vi "Init TS DAC Results File.vi"(8 "error in":errorcluster, 11 "Generic Test Stand in":refnum<class "Generic Test Stand.lvclass">) -> (0 "error out":errorcluster, 3 "Generic Test Stand out":refnum<class "Generic Test Stand.lvclass">)   [LabVIEW 2019, in "Generic Test Stand.lvclass"]
uses:
  Generic Test Stand.lvclass
  Generic Test Stand.lvclass/Generic Test Stand.ctl
  DAC/DAC.lvclass
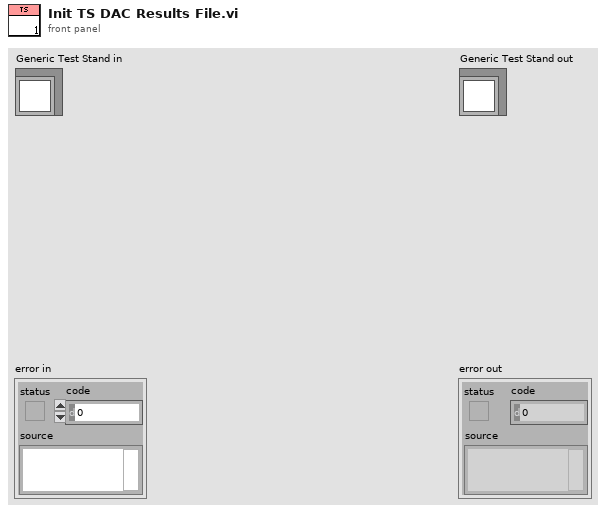
[diagram p1: front panel]
types:
  T1 = enum16{"open", "open or create", "create or replace", "create", "open (read-only)"}
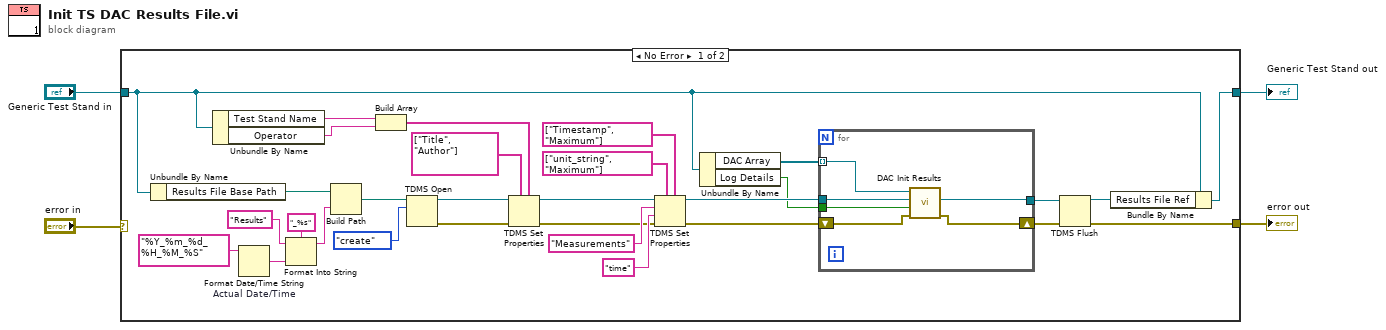
[diagram p0: block diagram]
diagram:
  n1 = case shown="No Error" "error in" {
    selector: "error in" -> [_ w42]
    tunnel: [w30 w42] -> w1
    tunnel: [w33 w41] -> w2
    tunnel: "Generic Test Stand in" -> [w21 w41]
    frame No Error {
      n2 = Unbundle By Name(w21) -> ("Results File Base Path"=w29:path)
      n3 = Unbundle By Name(w21) -> ("Test Stand Name"=w20:string, "Operator"=w19:string)
      n4 = Format Date/Time String "Actual Date/Time"(time format string (%c)="%Y_%m_%d_%H_%M_%S") -> (date/time string=w26:string)  [unwired: 2 in]
      n5 = Format Into String(format string="_%s", initial string="Results", w26) -> (resulting string=w24:string)  [unwired: 1 in, 1 out]
      n6 = Build Path(base path=w29, name or relative path=w24) -> (appended path=w23:path)
      n7 = Build Array(w20, w19) -> (w16:string[])
      n8 = TDMS Open(10:T1."create" ("operation (0:open)"), 11:w23) -> (0:w15:errorcluster, 3:w18:refnum<k34>)  [unwired: 5 in]
      n9 = TDMS Set Properties(5:w16, 7:string[] ["Title", "Author"] ("property names"), 8:w15, 11:w18) -> (0:w9:errorcluster, 3:w10:refnum<k34>)  [unwired: 2 in, 2 out]
      n10 = TDMS Set Properties(5:string[] ["Timestamp", "Maximum"] ("property names"), 7:string[] ["unit_string", "Maximum"] ("property names"), 8:w9, 9:"time" ("channel name"), 10:"Measurements" ("group name in (Untitled)"), 11:w10) -> (0:w8:errorcluster, 3:w7:refnum<k34>)  [unwired: 2 out]
      n11 = Unbundle By Name(w21) -> ("DAC Array"=w34:refnum<class "DAC.lvclass">[], "Log Details"=w5:bool)
      n12 = for {
        tunnel: w34 -> [w36] mode=indexing
        shift-right: [w38] -> w31
        shift-left: w8 -> [w39]
        tunnel: w7 -> [w40]
        tunnel: [w37] -> w6
        tunnel: w5 -> [w35]
        n13 = call-dynamic "DAC Init Results.vi"("error in"=w39, "Log Details?"=w35, "tdms file"=w40, "DAC in"=w36) -> ("error out"=w38:errorcluster, "tdms file out"=w37:refnum<k34>)  [unwired: 6 in]
      }
      n14 = TDMS Flush(4:w31, 7:w6) -> (0:w30:errorcluster, 3:w32:refnum<k34>)
      n15 = Bundle By Name(cluster=w21, "Results File Ref"=w32) -> (w33:refnum<class "Generic Test Stand.lvclass">)
    }
    frame Error {
    }
  }
  "error out" <- w1
  "Generic Test Stand out" <- w2
